vi "Pitchpack Commands.vi"(8 "error in (no error)":errorcluster, 11 "Command Queue In":refnum<queue>) -> (0 "error out":errorcluster, 3 "Command Queue Out":refnum<queue>)   [LabVIEW 2016]
uses:
  Message Format.ctl
  StateDef_generic.ctl
  <vilib>/addons/zeromq/socket_type.ctl
  <vilib>/addons/zeromq/socket_options.ctl
  <vilib>/addons/zeromq/zmq_context.lvclass
  <vilib>/addons/zeromq/zmq_socket.lvclass
  <vilib>/addons/zeromq/zeromq.lvlib
panel:
  out "data":string
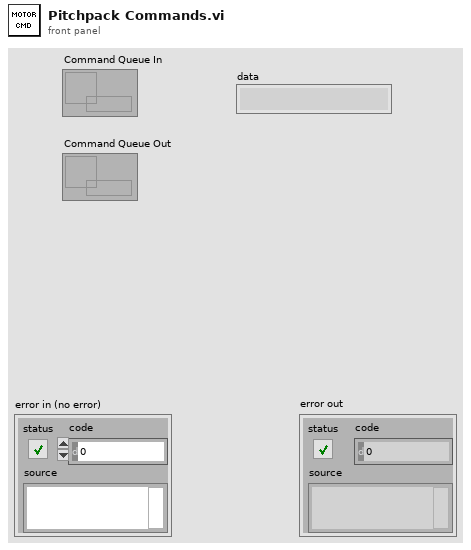
[diagram p1: front panel]
types:
  T1 = typedef "StateDef_generic.ctl" = enum16{"Initialize", "Running", "Exit"}
  T2 = typedef "zeromq.lvlib/socket_options.ctl" = enum8{"NONE", "ZMQ_HWM", "<2>", "ZMQ_SWAP", "ZMQ_AFFINITY", "ZMQ_IDENTITY", "ZMQ_SUBSCRIBE", "ZMQ_UNSUBSCRIBE", "ZMQ_RATE", "ZMQ_RECOVERY_IVL", "ZMQ_MCAST_LOOP", "ZMQ_SNDBUF", "ZMQ_RCVBUF", "ZMQ_RCVMORE", "ZMQ_FD", "ZMQ_EVENTS", "ZMQ_TYPE", "ZMQ_LINGER", "ZMQ_RECONNECT_IVL", "ZMQ_BACKLOG", "ZMQ_RECOVERY_IVL_MSEC", "ZMQ_RECONNECT_IVL_MAX", "ZMQ_MAXMSGSIZE", "ZMQ_SNDHWM", "ZMQ_RCVHWM", "ZMQ_MULTICAST_HOPS", "<26>", "ZMQ_RCVTIMEO", "ZMQ_SNDTIMEO", "<29>", "<30>", "ZMQ_IPV4ONLY", "ZMQ_LAST_ENDPOINT", "ZMQ_ROUTER_MANDATORY", "ZMQ_TCP_KEEPALIVE", "ZMQ_TCP_KEEPALIVE_CNT", "ZMQ_TCP_KEEPALIVE_IDLE", "ZMQ_TCP_KEEPALIVE_INTVL", "ZMQ_TCP_ACCEPT_FILTER", "ZMQ_DELAY_ATTACH_ON_CONNECT", "ZMQ_XPUB_VERBOSE"}
  T3 = typedef "zeromq.lvlib/socket_type.ctl" = enum8{"ZMQ_PAIR", "ZMQ_PUB", "ZMQ_SUB", "ZMQ_REQ", "ZMQ_REP", "ZMQ_DEALER", "ZMQ_ROUTER", "ZMQ_PULL", "ZMQ_PUSH", "ZMQ_XPUB", "ZMQ_XSUB"}
  T4 = typedef "Message Format.ctl" = cluster{"header":string, "data":variant}
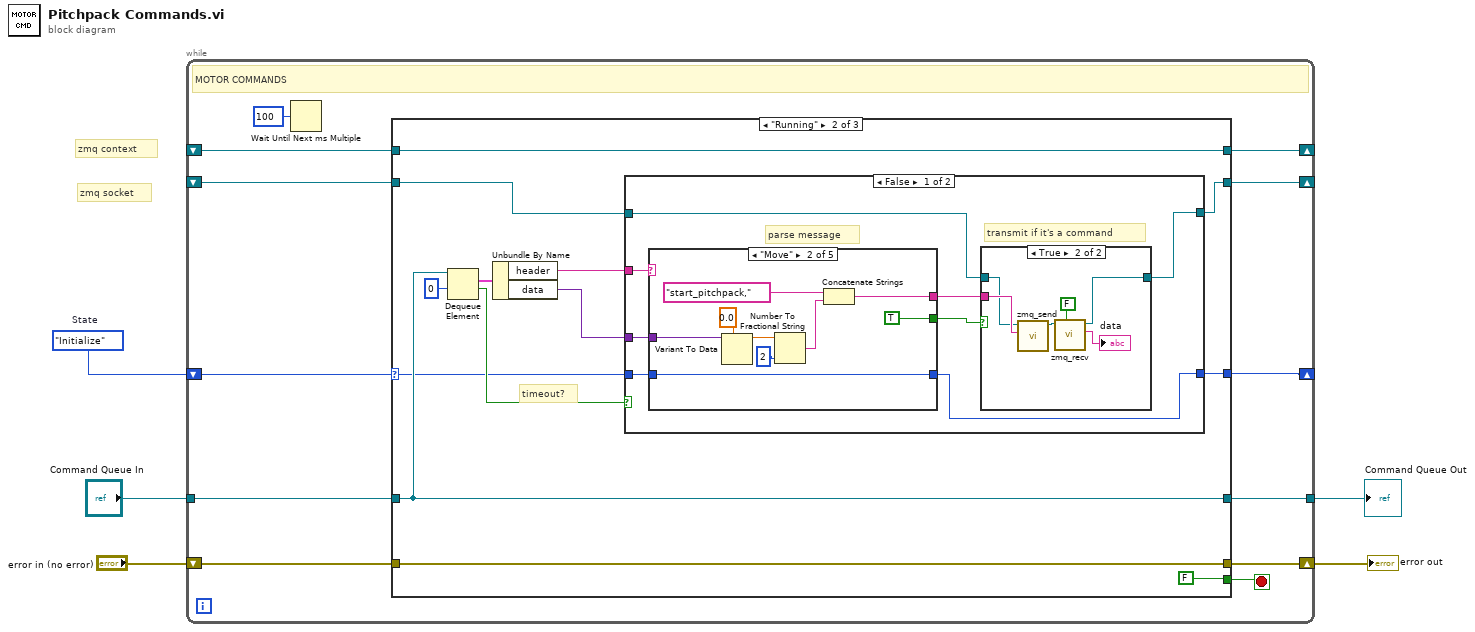
[diagram p0: block diagram]
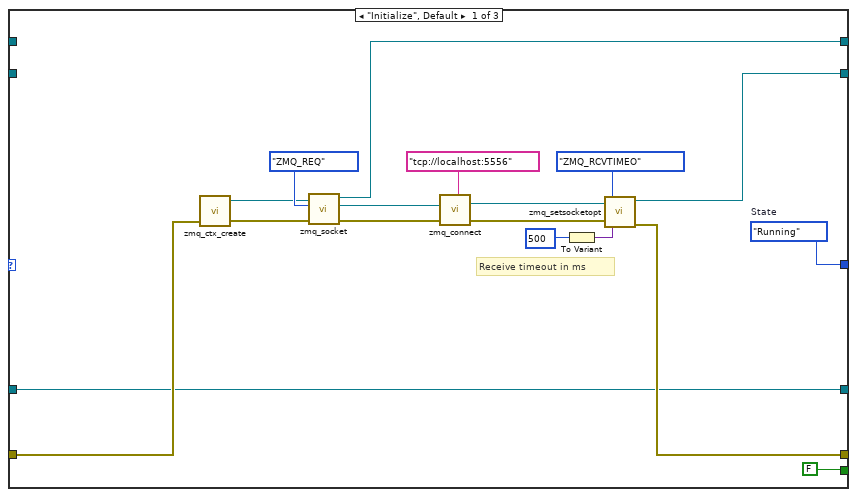
[diagram p2: hidden frame]
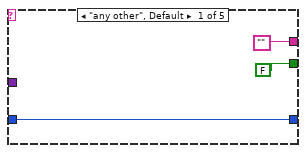
[diagram p4: hidden frame]
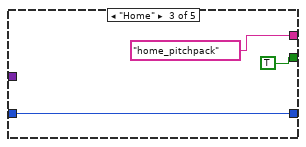
[diagram p5: hidden frame]
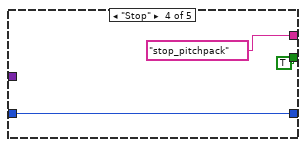
[diagram p6: hidden frame]
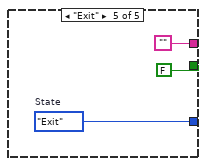
[diagram p7: hidden frame]
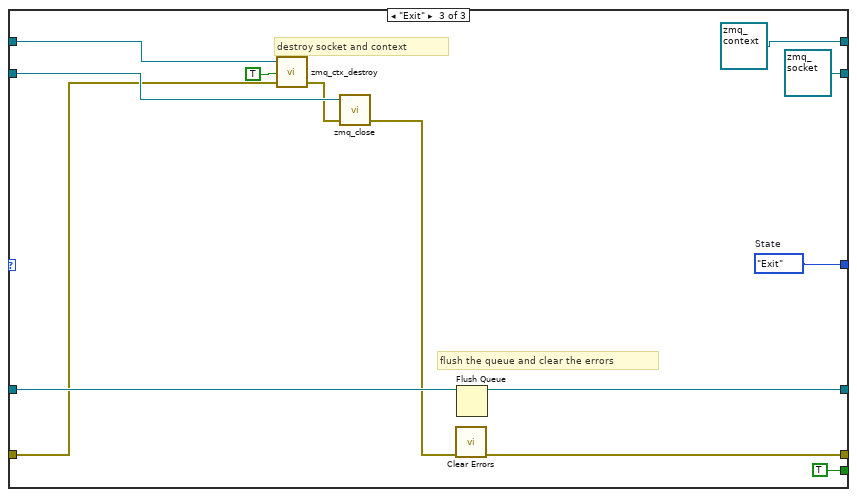
[diagram p9: hidden frame]
diagram:
  w3 = StateDef_generic."Initialize"  # State
  # "zmq socket"
  # "zmq context"
  n1 = while {
    shift-right: [w17] -> w2
    shift-left: "error in (no error)" -> [w10]
    shift-right: [w15] -> _
    shift-left: _ -> [w14]
    shift-right: [w13] -> _
    shift-left: _ -> [w12]
    tunnel: "Command Queue In" -> [w8]
    shift-right: [w9] -> _
    shift-left: w3 -> [w11]
    tunnel: [w6] -> w1
    stop <- w7 stop-if-true
    # "MOTOR COMMANDS"
    n2 = Wait Until Next ms Multiple(millisecond multiple=u32 100) -> ()  [unwired: 1 out]
    n3 = case shown="\"Running\"" w11 {
      selector: w11 -> [_ w40 _]
      tunnel: [w35 w36 w90] -> w17
      tunnel: [w34 w39 refnum<class "zmq_socket.lvclass"> refnum ("socket out")] -> w15
      tunnel: w14 -> [_ w41 w96]
      tunnel: [w23 w48 refnum<class "zmq_context.lvclass"> refnum ("context out")] -> w13
      tunnel: w12 -> [_ w48 w99]
      tunnel: w10 -> [w24 w36 w89]
      tunnel: [w20 w38 w97] -> w9
      tunnel: w8 -> [w18 w45 w93]
      tunnel: [FALSE FALSE TRUE] -> w7
      tunnel: [w18 w45 w87] -> w6
      frame "Initialize", Default {
        w20 = StateDef_generic."Running"  # State
        # "Receive timeout in ms"
        n4 = call <vilib>:"zmq_ctx_create.vi"("error in"=w24) -> ("error out"=w28:errorcluster, "context out"=w25:refnum<class "zmq_context.lvclass">)  [unwired: 3 in]
        n5 = call <vilib>:"zmq_socket.vi"("error in"=w28, "socket type"=socket_type."ZMQ_REQ", "context in"=w25) -> ("error out"=w21:errorcluster, "socket out"=w26:refnum<class "zmq_socket.lvclass">, "context out"=w23:refnum<class "zmq_context.lvclass">)  [unwired: 2 in]
        n6 = call <vilib>:"zmq_connect.vi"("error in"=w21, "endpoint"="tcp://localhost:5556", "socket in"=w26) -> ("error out"=w30:errorcluster, "socket out"=w22:refnum<class "zmq_socket.lvclass">)  [unwired: 1 in]
        n7 = To Variant(anything=500) -> (Variant=w33:variant)
        n8 = call <vilib>:"zmq_setsocketopt.vi"("error in"=w30, "value"=w33, "option"=socket_options."ZMQ_RCVTIMEO", "socket in"=w22) -> ("error out"=w35:errorcluster, "socket out"=w34:refnum<class "zmq_socket.lvclass">)  [unwired: 2 in]
      }
      frame "Running" {
        # "timeout?"
        n9 = Dequeue Element(queue=w45, timeout in ms (-1)=0) -> (element=w46:T4, timed out?=w44:bool)  [unwired: 1 in, 2 out]
        n10 = Unbundle By Name(w46) -> ("header"=w43:string, "data"=w42:variant)
        n11 = case shown="False" w44 {
          tunnel: w43 -> [w56 _]
          tunnel: w42 -> [w53 _]
          tunnel: w41 -> [w52 w85]
          tunnel: w40 -> [w51 w86]
          tunnel: [w50 w85] -> w39
          tunnel: [w49 w86] -> w38
          frame False {
            # "parse message"
            # "transmit if it's a command"
            n12 = case shown="\"Move\"" w56 {
              tunnel: [FALSE TRUE TRUE TRUE FALSE] -> w55
              tunnel: ["" w67 "home_pitchpack" "stop_pitchpack" ""] -> w54
              tunnel: w53 -> [_ w75 _ _ _]
              tunnel: w51 -> [w64 w73 w76 w79 _]
              tunnel: [w64 w73 w76 w79 w82] -> w49
              frame "any other", Default {
              }
              frame "Move" {
                n13 = Variant To Data(type=0.0, Variant=w75) -> (data=w71:dbl)  [unwired: 1 in, 1 out]
                n14 = Number To Fractional String(number=w71, precision (6)=i16 2 ("width (-)")) -> (F-format string=w68:string)  [unwired: 2 in]
                n15 = Concatenate Strings("start_pitchpack,", w68) -> (w67:string)
              }
              frame "Home" {
              }
              frame "Stop" {
              }
              frame "Exit" {
                w82 = StateDef_generic."Exit"  # State
              }
            }
            n16 = case shown="True" w55 {
              tunnel: w54 -> [_ w61]
              tunnel: w52 -> [w57 w59]
              tunnel: [w57 w58] -> w50
              frame False {
              }
              frame True {
                n17 = call <vilib>:"zmq_send.vi"("data"=w61, "socket in"=w59) -> ("socket out"=w63:refnum<class "zmq_socket.lvclass">)  [unwired: 5 in, 1 out]
                n18 = call <vilib>:"zmq_recv.vi"("no block? (F)"=FALSE, "socket in"=w63) -> ("data"=→"data":string, "socket out"=w58:refnum<class "zmq_socket.lvclass">)  [unwired: 3 in, 3 out]
              }
            }
          }
          frame True {
          }
        }
      }
      frame "Exit" {
        w97 = StateDef_generic."Exit"  # State
        # "flush the queue and clear the errors"
        # "destroy socket and context"
        n19 = call <vilib>:"zmq_ctx_destroy.vi"("error in"=w89, "reap? (F)"=TRUE, "context in"=w99) -> ("error out"=w91:errorcluster)  [unwired: 2 in]
        n20 = call <vilib>:"zmq_close.vi"("error in"=w91, "socket"=w96) -> ("error out"=w88:errorcluster)  [unwired: 3 in]
        n21 = call <vilib>:"Clear Errors.vi"("error in (no error)"=w88) -> ("error out"=w90:errorcluster)  [unwired: 5 in, 1 out]
        n22 = Flush Queue(queue=w93) -> (queue out=w87:refnum<queue>)  [unwired: 1 in, 2 out]
      }
    }
  }
  "error out" <- w2
  "Command Queue Out" <- w1
